vi "Single recall.vi"(2 "Min limit":dbl format="%.6f", 3 "Caption":string, 4 "Max limit":dbl format="%.6f", 5 "Input value":dbl format="%.6f") -> (0 "Continue? (T=yes)":bool=TRUE, 1 "Input value":dbl format="%.2f")   [LabVIEW 2010]
panel:
  in  "Exit":bool
  in  "OK":bool
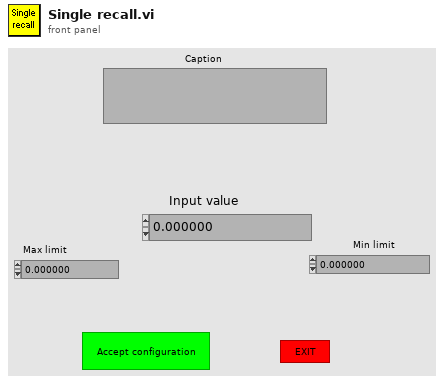
[diagram p1: front panel]
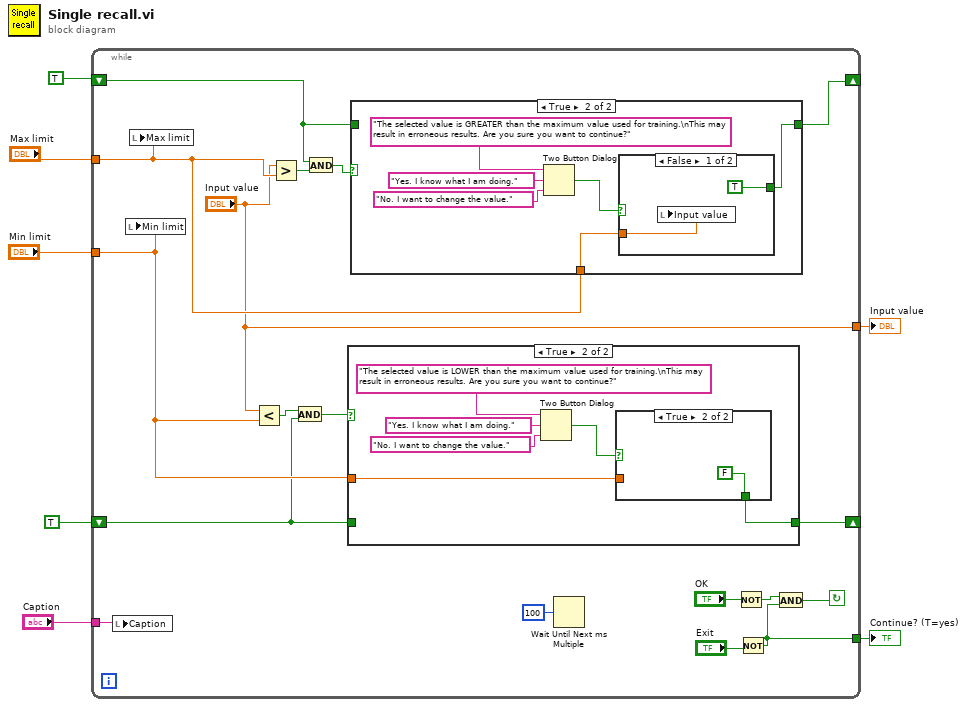
[diagram p0: block diagram]
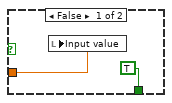
[diagram p3: hidden frame]
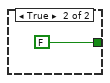
[diagram p5: hidden frame]
diagram:
  n1 = while {
    tunnel: ["Input value"] -> w1
    shift-left: TRUE -> [w9]
    shift-right: [w12] -> _
    shift-left: TRUE -> [w13]
    shift-right: [w14] -> _
    tunnel: "Min limit" -> [w17]
    tunnel: "Max limit" -> [w18]
    tunnel: "Caption" -> [w19]
    tunnel: [w21] -> w7
    stop <- w22 continue-if-true
    n2 = local write "Caption"(w19) -> ()
    n3 = local write "Min limit"(w17) -> ()
    n4 = local write "Max limit"(w18) -> ()
    n5 = Less?(x="Input value", y=w17) -> (x < y?=w11:bool)
    n6 = Greater?(x="Input value", y=w18) -> (0:w16:bool)
    n7 = And(x=w11, y=w9) -> (x .and. y?=w10:bool)
    n8 = And(x=w13, y=w16) -> (x .and. y?=w15:bool)
    n9 = case shown="True" w10 {
      tunnel: w17 -> [_ w28]
      tunnel: [w26 w27] -> w12
      tunnel: w9 -> [w26 _]
      frame False {
      }
      frame True {
        n10 = Two Button Dialog(message="The selected value is LOWER than the maximum value used for training.\nThis may result in erroneous results. Are you sure you want to continue?", 1:"No. I want to change the value." ("T button name (\"OK\")"), 2:"Yes. I know what I am doing." ("T button name (\"OK\")")) -> (T button?=w29:bool)
        n11 = case shown="True" w29 {
          tunnel: w28 -> [w34 _]
          tunnel: [TRUE FALSE] -> w27
          frame False {
            n12 = local write "Input value"(w34) -> ()
          }
          frame True {
          }
        }
      }
    }
    n13 = case shown="True" w15 {
      tunnel: w18 -> [_ w38]
      tunnel: [w36 w37] -> w14
      tunnel: w13 -> [w36 _]
      frame False {
      }
      frame True {
        n14 = Two Button Dialog(message="The selected value is GREATER than the maximum value used for training.\nThis may result in erroneous results. Are you sure you want to continue?", 1:"No. I want to change the value." ("T button name (\"OK\")"), 2:"Yes. I know what I am doing." ("T button name (\"OK\")")) -> (T button?=w39:bool)
        n15 = case shown="False" w39 {
          tunnel: w38 -> [w44 _]
          tunnel: [TRUE FALSE] -> w37
          frame False {
            n16 = local write "Input value"(w44) -> ()
          }
          frame True {
          }
        }
      }
    }
    n17 = Wait Until Next ms Multiple(millisecond multiple=u32 100) -> ()  [unwired: 1 out]
    n18 = Not(x="OK") -> (.not. x?=w24:bool)
    n19 = Not(x="Exit") -> (.not. x?=w21:bool)
    n20 = And(x=w24, y=w21) -> (x .and. y?=w22:bool)
  }
  "Continue? (T=yes)" <- w7
  "Input value" <- w1
